vi "DeviationMeasurement.vi"(0 "Connection Cluster in":T1, 5 "Wanted thickness":dbl, 7 "Refractive Index":dbl, 9 "Peak position":dbl, 11 "Thickness range":dbl, 12 "Compensation factor":dbl) -> (4 "Connection Cluster out":T1, 6 "Lens thickness right":dbl, 8 "Thickness right in range?":bool, 10 "Lens thickness left":dbl, 13 "Lens thickness average":dbl, 14 "Lens thickness in range? average":bool, 15 "Thickness left in range?":bool)   [LabVIEW 2013]
uses:
  Global.vi
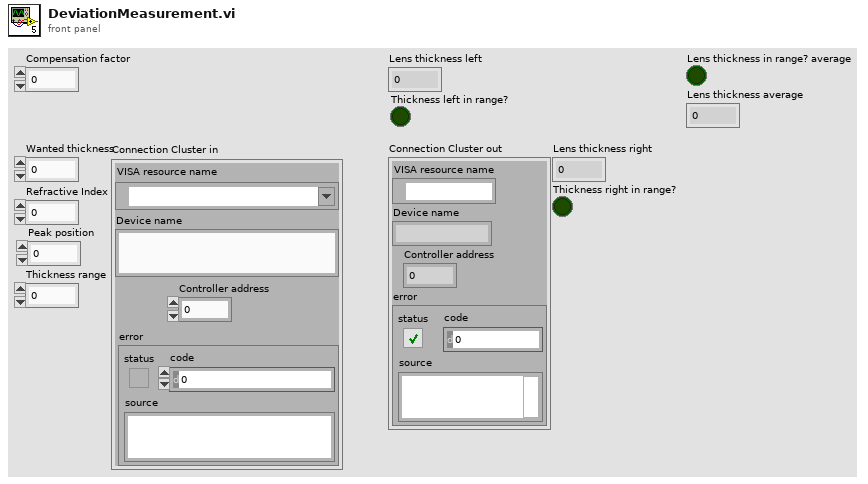
[diagram p1: front panel]
types:
  T1 = cluster{"VISA resource name":refnum<visa-resource-name>, "Device name":string, "Controller address":i32, "error":errorcluster}
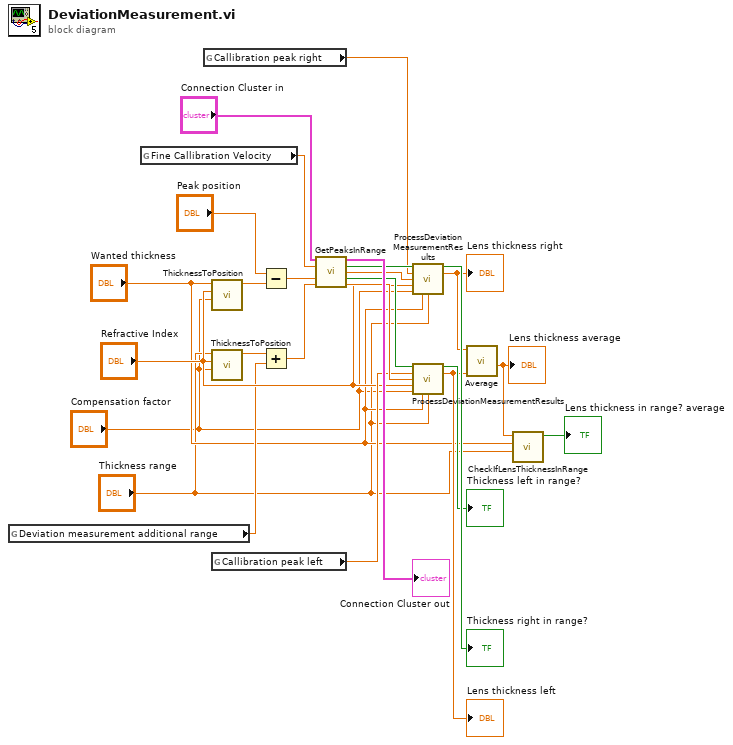
[diagram p0: block diagram]
diagram:
  n1 = global read "Global.vi" "Deviation measurement additional range"() -> (w8:dbl)
  n2 = global read "Global.vi" "Fine Callibration Velocity"() -> (w24:dbl)
  n3 = global read "Global.vi" "Callibration peak right"() -> (w17:dbl)
  n4 = call "ThicknessToPosition.vi"("Compensation factor"="Compensation factor", "Refractive Index"="Refractive Index", "Thickness"="Wanted thickness") -> ("Position"=w21:dbl)  [unwired: 8 in]
  n5 = call "ThicknessToPosition.vi"("Compensation factor"="Compensation factor", "Refractive Index"="Refractive Index", "Thickness"="Thickness range") -> ("Position"=w10:dbl)  [unwired: 8 in]
  n6 = global read "Global.vi" "Callibration peak left"() -> (w13:dbl)
  n7 = Subtract(x="Peak position", y=w21) -> (x-y=w20:dbl)
  n8 = Add(x=w10, y=w8) -> (x+y=w9:dbl)
  n9 = call "GetPeaksInRange.vi"("Connection Cluster in"="Connection Cluster in", "Fine Callibration Velocity 2"=w24, "Start Position"=w20, "Fine range"=w9) -> ("Connection Cluster out"=→"Connection Cluster out":T1, "Peak detected? right"=w19:bool, "Peak (right)"=w16:dbl, "Peak detected? left"=w15:bool, "Peak (left)"=w14:dbl)  [unwired: 7 in]
  n10 = call "ProcessDeviationMeasurementResults.vi"("Peak detected?"=w19, "Callibration Peak Position"=w17, "Measurement Peak Position"=w16, "Refractive index"="Refractive Index", "Compensation factor"="Compensation factor", "Wanted thickness"="Wanted thickness", "Thickness range"="Thickness range") -> ("Lens thickness in range?"=→"Thickness right in range?":bool, "Lens thickness"=w7:dbl)  [unwired: 7 in]
  "Lens thickness right" <- w7
  n11 = call "ProcessDeviationMeasurementResults.vi"("Peak detected?"=w15, "Callibration Peak Position"=w13, "Measurement Peak Position"=w14, "Refractive index"="Refractive Index", "Compensation factor"="Compensation factor", "Wanted thickness"="Wanted thickness", "Thickness range"="Thickness range") -> ("Lens thickness in range?"=→"Thickness left in range?":bool, "Lens thickness"=w6:dbl)  [unwired: 7 in]
  "Lens thickness left" <- w6
  n12 = call "Average.vi"("y"=w6, "x"=w7) -> ("Average"=w5:dbl)  [unwired: 9 in]
  "Lens thickness average" <- w5
  n13 = call "CheckIfLensThicknessInRange.vi"("Thickness range"="Thickness range", "Wanted thickness"="Wanted thickness", "Lens thickness"=w5) -> ("Lens thickness in range?"=→"Lens thickness in range? average":bool)  [unwired: 8 in]
